vi "New TextDocument.vi"(7 "ooWriter":refnum<class "ooWriter.lvclass">, 8 "error in (no error)":errorcluster, 10 "template (empty)":path) -> (0 "error out":errorcluster, 3 "ooWriter out":refnum<class "ooWriter.lvclass">)   [LabVIEW 2009, in "ooWriter.lvclass"]
uses:
  ooWriter.lvclass
  C:/Projets/LAVAG/OpenOfficeRGT/AODL/DLLs/AODL.dll
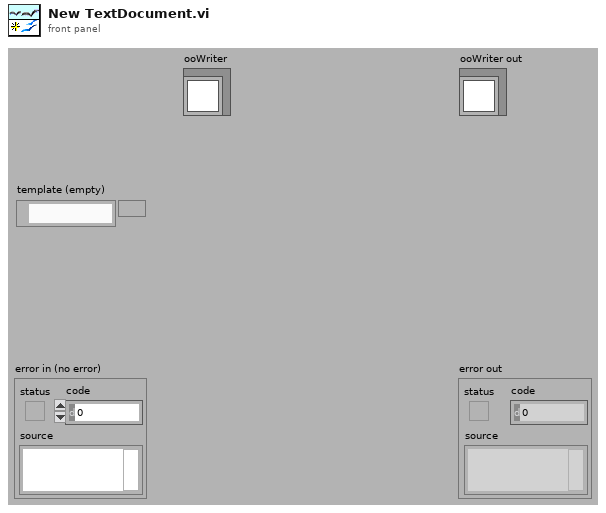
[diagram p1: front panel]
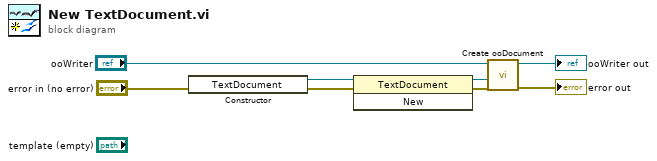
[diagram p0: block diagram]
diagram:
  n1 = constructor class="TextDocument"(error in="error in (no error)") -> (reference out=w8:refnum<k24>, error out=w6:errorcluster)  [unwired: 2 in, 1 out]
  n2 = invoke class="TextDocument" method="New"(reference=w8, error in=w6) -> (reference out=w7:refnum<k24>, error out=w5:errorcluster)  [unwired: 1 in, 1 out]
  n3 = call-dynamic "Create ooDocument.vi"("error in (no error)"=w5, "Document"=w7, "ooDocument in"="ooWriter") -> ("error out"=→"error out":errorcluster, "ooDocument out"=→"ooWriter out":refnum<class "ooWriter.lvclass">)  [unwired: 7 in]
